vi "Configure Band Selector Visibility.vi"(8 "error in (no error)":errorcluster, 10 "Number of Bands in":u8, 11 "Enum Refnum":refnum<vi>[](array[refnum])) -> (0 "error out":errorcluster, 2 "Number of Bands out":u8)   [LabVIEW 2018, in "Front Panel Inteface.lvlib"]
uses:
  Front Panel Inteface.lvlib
  Digit--control.ctl
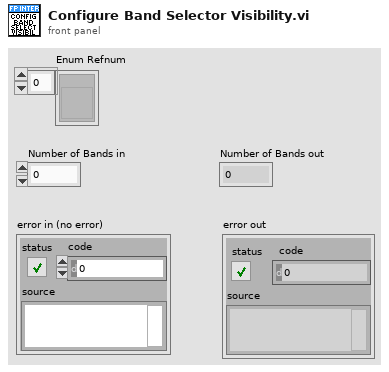
[diagram p1: front panel]
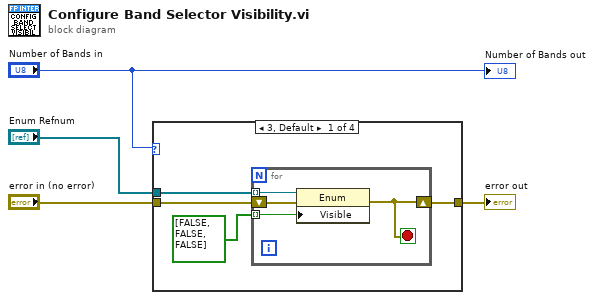
[diagram p0: block diagram]
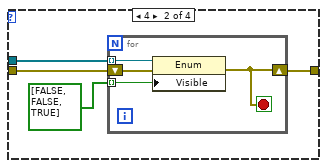
[diagram p2: hidden frame]
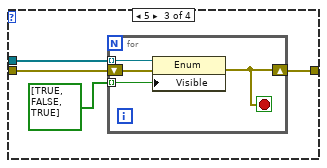
[diagram p3: hidden frame]
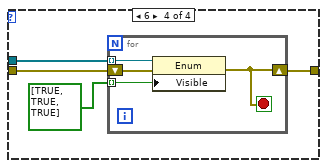
[diagram p4: hidden frame]
diagram:
  n1 = case shown="3, Default" "Number of Bands in" {
    tunnel: "error in (no error)" -> [w8 w13 w21 w29]
    tunnel: [w7 w15 w23 w31] -> w2
    tunnel: "Enum Refnum" -> [w5 w14 w22 w30]
    frame 3, Default {
      n2 = for {
        shift-right: [w11] -> w7
        shift-left: w8 -> [w12]
        tunnel: bool[] [FALSE, FALSE, FALSE] -> [w9] mode=indexing
        tunnel: w5 -> [w10] mode=indexing
        stop <- w11 stop-if-true
        n3 = property class="Enum"(reference=w10, error in=w12, "Visible"=w9) -> (error out=w11:errorcluster)  [unwired: 1 out]
      }
    }
    frame 4 {
      n4 = for {
        shift-right: [w19] -> w15
        shift-left: w13 -> [w20]
        tunnel: bool[] [FALSE, FALSE, TRUE] -> [w18] mode=indexing
        tunnel: w14 -> [w17] mode=indexing
        stop <- w19 stop-if-true
        n5 = property class="Enum"(reference=w17, error in=w20, "Visible"=w18) -> (error out=w19:errorcluster)  [unwired: 1 out]
      }
    }
    frame 5 {
      n6 = for {
        shift-right: [w27] -> w23
        shift-left: w21 -> [w28]
        tunnel: bool[] [TRUE, FALSE, TRUE] -> [w26] mode=indexing
        tunnel: w22 -> [w25] mode=indexing
        stop <- w27 stop-if-true
        n7 = property class="Enum"(reference=w25, error in=w28, "Visible"=w26) -> (error out=w27:errorcluster)  [unwired: 1 out]
      }
    }
    frame 6 {
      n8 = for {
        shift-right: [w35] -> w31
        shift-left: w29 -> [w36]
        tunnel: bool[] [TRUE, TRUE, TRUE] -> [w34] mode=indexing
        tunnel: w30 -> [w33] mode=indexing
        stop <- w35 stop-if-true
        n9 = property class="Enum"(reference=w33, error in=w36, "Visible"=w34) -> (error out=w35:errorcluster)  [unwired: 1 out]
      }
    }
  }
  "error out" <- w2
  "Number of Bands out" <- "Number of Bands in"
